vi "Ex6.vi"() -> ()   [LabVIEW 2018]
uses:
  Global 1.vi
panel:
  in  "stop":bool
  in  "OK Button":bool
  out "Boolean 2":bool
  out "Boolean":bool
  out "Numeric":dbl
  in  "Knob 3":i8(knob) min=0 max=9 scale=0.0..9.0
  in  "Knob 2":i8(knob) min=0 max=9 scale=0.0..9.0
  in  "Knob":i8(knob) min=0 max=9 scale=0.0..9.0
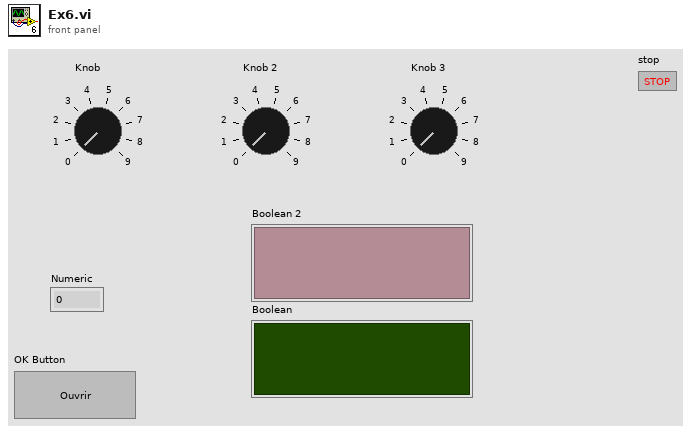
[diagram p1: front panel]
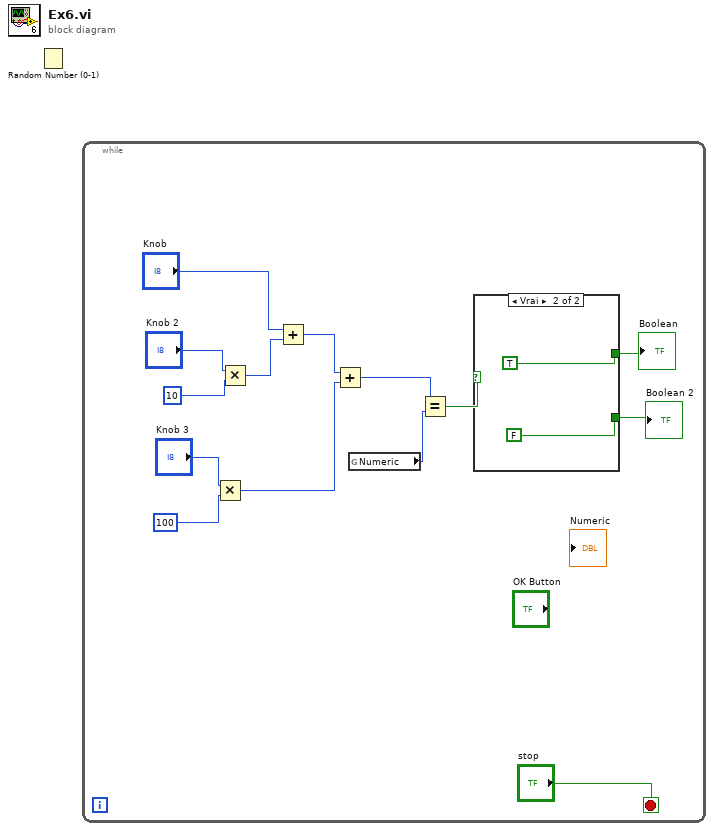
[diagram p0: block diagram]
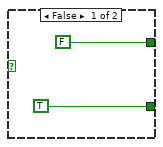
[diagram p2: hidden frame]
diagram:
  n1 = Random Number (0-1)() -> ()  [unwired: 1 out]
  n2 = while {
    stop <- "stop" stop-if-true
    n3 = Multiply(x="Knob 3", y=100) -> (x*y=w6:i32)
    n4 = Multiply(x="Knob 2", y=10) -> (x*y=w11:i32)
    n5 = Add(x="Knob", y=w11) -> (x+y=w7:i32)
    n6 = Add(x=w7, y=w6) -> (x+y=w5:i32)
    n7 = global read "Global 1.vi" "Numeric"() -> (w4:i16)
    n8 = Equal?(x=w5, y=w4) -> (x = y?=w1:bool)
    n9 = case shown="Vrai" w1 {
      tunnel: [FALSE ("Boolean 2") TRUE ("Boolean")] -> w3
      tunnel: [TRUE ("Boolean") FALSE ("Boolean 2")] -> w2
      frame False {
      }
      frame True {
      }
    }
    "Boolean" <- w3
    "Boolean 2" <- w2
  }
